vi "Configure Digital Output IQ Data.vi"(8 "error in (no error)":errorcluster, 9 "Q Gain (100 %)":dbl=100.0, 10 "I Gain (100 %)":dbl=100.0, 11 "VISA resource name":refnum<visa-resource-name>) -> (0 "error out":errorcluster, 3 "VISA resource name out":refnum<visa-resource-name>)   [LabVIEW 2018, in "Agilent PSG MXG Series.lvlib"]
doc: "Configures I and Q data for digital output data.\n\n<b>Note:</b>\nIt is only valid in N5172B/82B with <b>Option 003</b> or <b>Option 004</b> or <b>Option both</b>."
uses:
  Agilent PSG MXG Series.lvlib
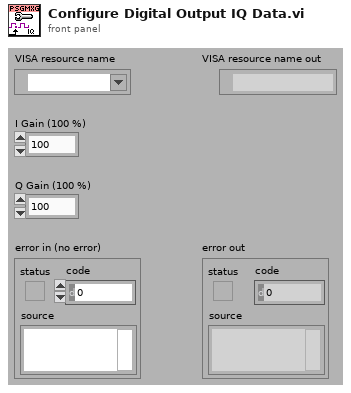
[diagram p1: front panel]
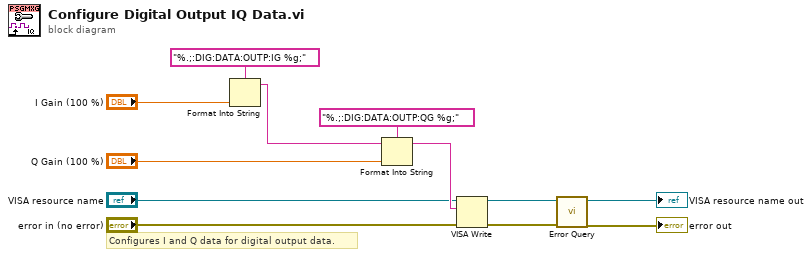
[diagram p0: block diagram]
diagram:
  # "Configures I and Q data for digital output data."
  n1 = Format Into String(format string="%.;:DIG:DATA:OUTP:IG %g;", "I Gain (100 %)") -> (resulting string=w10:string)  [unwired: 2 in, 1 out]
  n2 = Format Into String(format string="%.;:DIG:DATA:OUTP:QG %g;", initial string=w10, "Q Gain (100 %)") -> (resulting string=w7:string)  [unwired: 1 in, 1 out]
  n3 = VISA Write(VISA resource name="VISA resource name", write buffer=w7, error in (no error)="error in (no error)") -> (VISA resource name out=w4:refnum<visa-resource-name>, error out=w3:errorcluster)  [unwired: 1 out]
  n4 = call "Error Query.vi"("error in (no error)"=w3, "VISA resource name"=w4) -> ("error out"=→"error out":errorcluster, "VISA resource name out"=→"VISA resource name out":refnum<visa-resource-name>)  [unwired: 6 in, 2 out]
